vi "set Data Write.vi"(6 "data":u32, 7 "data_pos":u16, 8 "error in (no error)":errorcluster, 9 "data_length":u16, 10 "protocol_version":i32, 11 "port_num":i32) -> (0 "error out":errorcluster)   [LabVIEW 2022 SP3, in "dxl.lvlib"]
doc: "WINDECLSPEC void setDataWrite (int port_num, int protocol_version, uint16_t data_length, uint16_t data_pos, uint32_t data);"
uses:
  dxl.lvlib
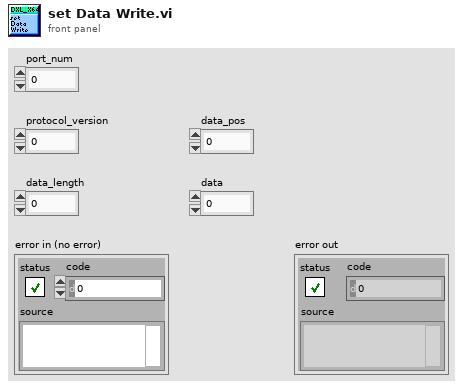
[diagram p1: front panel]
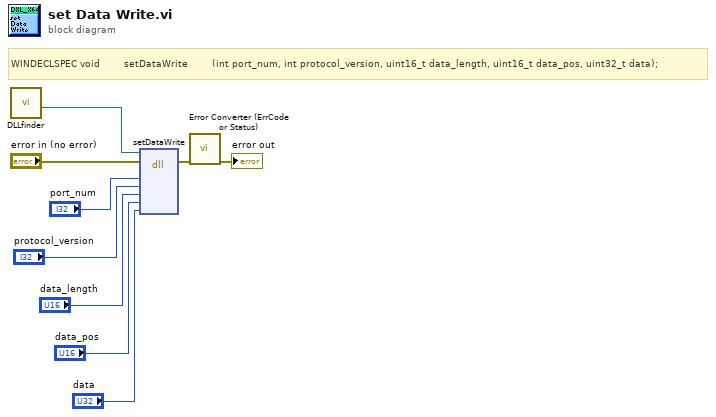
[diagram p0: block diagram]
diagram:
  # "WINDECLSPEC void        setDataWrite        (int port_num, int protocol_version, uint16_t data_length, uint16_t data_pos, uint32_t data);"
  n1 = call "DLLfinder.vi"() -> ("File Path"=w1:path)  [unwired: 11 in]
  n2 = dll-call lib="C:/EnFlo_Software/ADAM Serial/Instrument drivers/Dynamixel/2nd attempt/Library/dxl_x64_c.*" fn="setDataWrite"(path in=w1, error in="error in (no error)", "port_num"="port_num", "protocol_version"="protocol_version", "data_length"="data_length", "data_pos"="data_pos", "data"="data") -> (error out=w3:errorcluster)  [unwired: 7 in, 1 out]
  n3 = call "Error Converter (ErrCode or Status).vi"("error in (no error)"=w3) -> ("error out"=→"error out":errorcluster)  [unwired: 10 in]
